vi "TCP_test.vi"(10 "Mode":dbl, 11 "Array":dbl[](array[numeric])) -> (3 "Numeric":dbl)   [LabVIEW 2020]
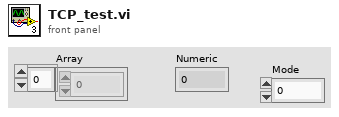
[diagram p1: front panel]
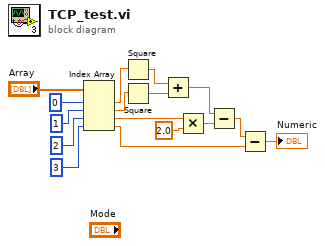
[diagram p0: block diagram]
diagram:
  n1 = Index Array(array="Array", index #1=0 ("index"), index #2=1 ("index"), index #3=2 ("index"), index #4=3 ("index")) -> (element #1=w5:dbl, element #2=w6:dbl, element #3=w10:dbl, element #4=w13:dbl)
  n2 = Square(x=w5) -> (x^2=w7:dbl)
  n3 = Square(x=w6) -> (x^2=w8:dbl)
  n4 = Add(x=w7, y=w8) -> (x+y=w11:dbl)
  n5 = Multiply(x=w10, y=2.0) -> (x*y=w12:dbl)
  n6 = Subtract(x=w11, y=w12) -> (x-y=w14:dbl)
  n7 = Subtract(x=w14, y=w13) -> (x-y=→"Numeric":dbl)
